vi "ProposedTargets.vi"(1 "Contol\nPoint\nSuffix":T3, 2 "Value":dbl, 3 "Type":i32, 4 "Geometry":i32) -> (0 "Target":T1={"LBCB Number"=enum."LBCB1", "DOF Vectors"=enum."Dx", "Amount"=0.0})   [LabVIEW 2009]
uses:
  lib/NTCP Client/Control Point Suffix.ctl
  lib/MixedMode/Messages/Target.ctl
  lib/Data Access Objects/Metadata/LBCB Number.ctl
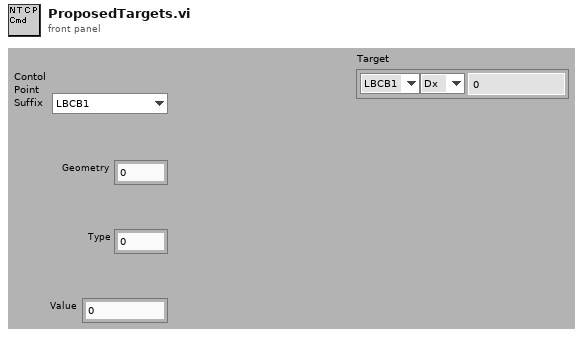
[diagram p1: front panel]
types:
  T1 = typedef "Target.ctl" = cluster{"LBCB Number":T2, "DOF Vectors":enum16{" ", "Dx", "Dy", "Dz", "Rx", "Ry", "Rz", "Fx", "Fy", "Fz", "Mx", "My", "Mz"}, "Amount":dbl}
  T2 = typedef "LBCB Number.ctl" = enum16{"LBCB1", "LBCB2"}
  T3 = typedef "Control Point Suffix.ctl" = enum16{"LBCB1", "LBCB2", "ExternalSensors"}
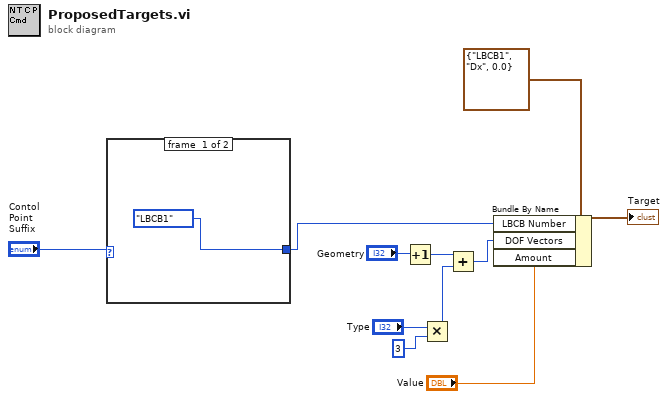
[diagram p0: block diagram]
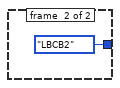
[diagram p2: hidden frame]
diagram:
  n1 = case shown="\"LBCB2\"" "Contol\nPoint\nSuffix" {
    tunnel: [LBCB_Number."LBCB1" ("LBCB Number") LBCB_Number."LBCB2" ("LBCB Number")] -> w1
    frame #0 {
    }
    frame #1 {
    }
  }
  n2 = Increment(x="Geometry") -> (x+1=w6:i32)
  n3 = Multiply(x="Type", y=3) -> (x*y=w5:i32)
  n4 = Add(x=w6, y=w5) -> (x+y=w4:i32)
  n5 = Bundle By Name(cluster=T1 {"LBCB Number"=enum."LBCB1", "DOF Vectors"=enum."Dx", "Amount"=0.0} ("Target"), "LBCB Number"=w1, "DOF Vectors"=w4, "Amount"="Value") -> (→"Target":T1)
